vi "Decode Single Line.vi"(11 "Line":string) -> (0 "Valve Action":T1, 1 "Valve ID":u32, 2 "Time":u32, 3 "Valid?":bool)   [LabVIEW 2015]
uses:
  Valve Action Enum.ctl
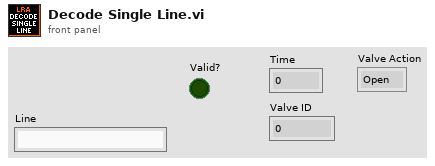
[diagram p1: front panel]
types:
  T1 = typedef "Valve Action Enum.ctl" = enum16{"Open", "Close"}
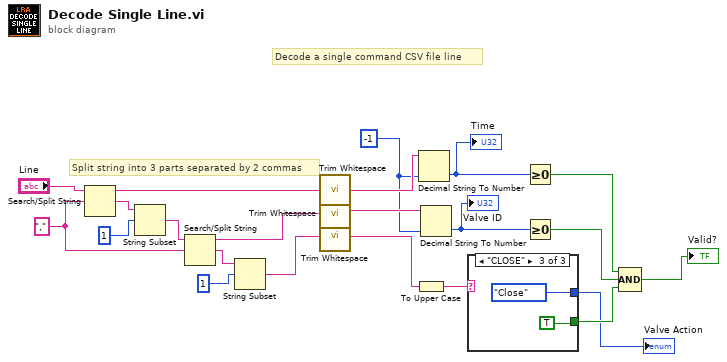
[diagram p0: block diagram]
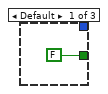
[diagram p2: hidden frame]
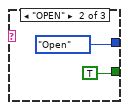
[diagram p3: hidden frame]
diagram:
  w5 = -1 ("Time")
  w19 = "," ("search string/char (-)")
  # "Split string into 3 parts separated by 2 commas"
  # "Decode a single command CSV file line"
  n1 = Search/Split String(string="Line", search string/char (-)=w19) -> (substring before match=w13:string, match + rest of string=w16:string)  [unwired: 1 in, 1 out]
  n2 = String Subset(string=w16, offset (0)=1) -> (substring=w20:string)  [unwired: 1 in]
  n3 = Search/Split String(string=w20, search string/char (-)=w19) -> (substring before match=w14:string, match + rest of string=w18:string)  [unwired: 1 in, 1 out]
  n4 = String Subset(string=w18, offset (0)=1) -> (substring=w15:string)  [unwired: 1 in]
  n5 = call <vilib>:"Trim Whitespace.vi"("string"=w13) -> ("trimmed string"=w12:string)  [unwired: 1 in]
  n6 = call <vilib>:"Trim Whitespace.vi"("string"=w14) -> ("trimmed string"=w11:string)  [unwired: 1 in]
  n7 = call <vilib>:"Trim Whitespace.vi"("string"=w15) -> ("trimmed string"=w10:string)  [unwired: 1 in]
  n8 = To Upper Case(1:w10) -> (0:w9:string)
  n9 = Decimal String To Number(string=w12, default (0L)=w5) -> (number=w3:i32)  [unwired: 1 in, 1 out]
  "Time" <- w3
  n10 = Decimal String To Number(string=w11, default (0L)=w5) -> (number=w4:i32)  [unwired: 1 in, 1 out]
  "Valve ID" <- w4
  n11 = case shown="\"CLOSE\"" w9 {
    tunnel: [_ Valve_Action_Enum."Open" Valve_Action_Enum."Close"] -> w6
    tunnel: [FALSE TRUE TRUE] -> w8
    frame Default {
    }
    frame "OPEN" {
    }
    frame "CLOSE" {
    }
  }
  "Valve Action" <- w6
  n12 = Greater Or Equal To 0?(x=w3) -> (x >= 0?=w2:bool)
  n13 = Greater Or Equal To 0?(x=w4) -> (x >= 0?=w1:bool)
  n14 = Compound Arithmetic op=AND(w2, w1, w8) -> (→"Valid?":bool)
